vi "Read PS Current.vi"(8 "error in":errorcluster, 11 "PS":refnum<visa-resource-name>) -> (0 "error out":errorcluster, 2 "Current Measurement":dbl format="%.2f")   [LabVIEW 2015]
uses:
  <instrlib>/BK Precision 178XB Series/BK Precision 178XB Series.lvlib
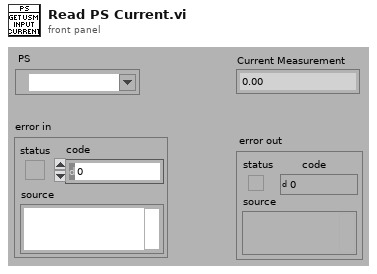
[diagram p1: front panel]
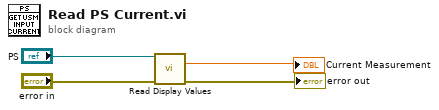
[diagram p0: block diagram]
diagram:
  n1 = call <instrlib>:"Read Display Values.vi"("VISA resource name"="PS", "error in (no error)"="error in") -> ("Terminal Output Current"=→"Current Measurement":dbl, "error out"=→"error out":errorcluster)  [unwired: 10 in, 2 out]
